vi "Load Firmware.vi"(8 "error in (no error)":errorcluster, 10 "Channels":u8[](array[numeric]), 11 "ID In":i32) -> (0 "error out":errorcluster, 2 "Results":i32[](array[numeric]), 3 "ID Out":i32)   [LabVIEW 2022 SP3, in "EClib functions.lvlib"]
doc: "This VI loads the kernel.bin and evetually the x100_01.txt files in the selected channels.\nThe firmware is loading only if necessary."
uses:
  EClib functions.lvlib
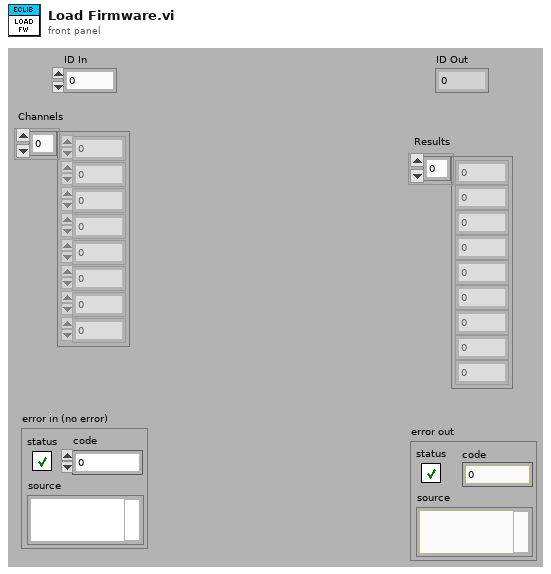
[diagram p1: front panel]
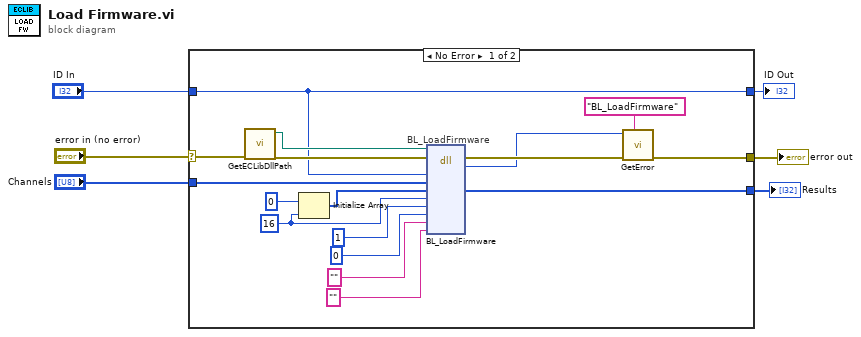
[diagram p0: block diagram]
diagram:
  n1 = case shown="No Error" "error in (no error)" {
    selector: "error in (no error)" -> [w13 w24]
    tunnel: [w14 w24] -> w6
    tunnel: "ID In" -> [w7 w25]
    tunnel: "Channels" -> [w10 _]
    tunnel: [w9 _] -> w2
    tunnel: [w7 w25] -> w1
    frame No Error {
      w20 = 16 ("dimension size")
      # "BL_LoadFirmware"
      n2 = call "GetECLibDllPath.vi"("error in (no error)"=w13) -> ("error out"=w12:errorcluster, "ECLibDLLPath"=w18:path)  [unwired: 9 in]
      n3 = Initialize Array(0 ("element"), w20) -> (w19:i32[])
      n4 = dll-call lib="?" fn="BL_LoadFirmware"(path in=w18, error in=w12, "arg0"=w7, "arg1"=w10, "arg3"=w19, "arg4"=w20, "arg6"=1, "arg5"=0, "arg7"="", "arg8"="") -> (error out=w11:errorcluster, "return type"=w8:i32, "arg3"=w9:i32[])  [unwired: 8 in, 1 out]
      n5 = call "GetError.vi"("DLLFunction"="BL_LoadFirmware", "error in"=w11, "code"=w8) -> ("error out"=w14:errorcluster)  [unwired: 8 in]
    }
    frame Error {
    }
  }
  "error out" <- w6
  "Results" <- w2
  "ID Out" <- w1
